vi "LV86_Min.vi"(0 "Constant":u8=1, 2 "Image 2":T1={"Width"=0, "Height"=0, "Depth"=-1, "data"=[], "Compressed data"=[], "Color table"=[], "Duration"=0, "Options"=0, "Timestamp"=0, "ID"=0, "Reserved"=0, "Dialogs"=0} {"Dialogs" format="%.0b"}, 3 "Image":T1 {"Dialogs" format="%.0b"}) -> (1 "Image Out":T1 {"Dialogs" format="%.0b"})   [LabVIEW 2024]
doc: "This VI adds two images pixel by pixel or a constant to one image. If <B>Image 2</B> is unwired, the <B>constant</B> is added to the image. (Does not work on a color image)"
uses:
  <userlib>/ImageProcessing/QTLIB_2595_LV86/QT_Image.ctl
panel:
  # "This VI adds two images pixel by pixel or a constant\n to one image.  If Image 2 is unwired, the constant \nis added to the image. (Does not work on a color image)"
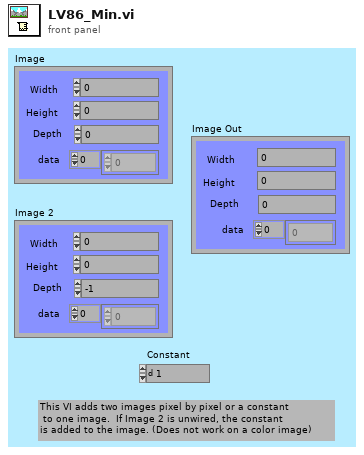
[diagram p1: front panel]
types:
  T1 = typedef "QT_Image.ctl" = cluster{"Width":i32, "Height":i32, "Depth":i32, "data":u8[], "Compressed data":u8[], "Color table":u32[], "Duration":i32, "Options":i32, "Timestamp":i32, "ID":i32, "Reserved":i32, "Dialogs":u32}
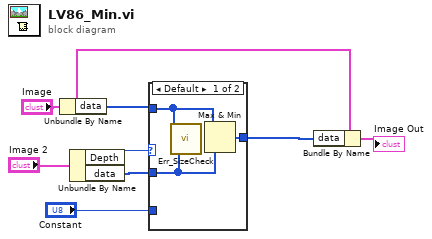
[diagram p0: block diagram]
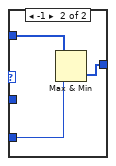
[diagram p2: hidden frame]
diagram:
  n1 = Unbundle By Name("Image") -> ("data"=w1:u8[])
  n2 = Unbundle By Name("Image 2") -> ("Depth"=w5:i32, "data"=w6:u8[])
  n3 = case shown="Default" w5 {
    tunnel: w1 -> [w11 w14]
    tunnel: "Constant" -> [_ w13]
    tunnel: [w9 w12] -> w2
    tunnel: w6 -> [w10 _]
    frame Default {
      n4 = call <userlib>:"Err_SizeCheck.vi"("data 2"=w10, "data"=w11) -> ()  [unwired: 2 out]
      n5 = Max & Min(x=w11, y=w10) -> (min(x,y)=w9:u8[])  [unwired: 1 out]
    }
    frame -1 {
      n6 = Max & Min(x=w14, y=w13) -> (min(x,y)=w12:u8[])  [unwired: 1 out]
    }
  }
  n7 = Bundle By Name(cluster="Image", "data"=w2) -> (→"Image Out":T1)
